vi "STARTUP.VI"() -> ()   [LabVIEW 2011]
uses:
  OIMENU.LLB/OIMenuItem1.ctl
panel:
  in  "ILM Setup Dialog":T1={"Go"=TRUE}
  in  "Array of VI's to open automatically on startup.\nCreate the list you require and save it using\nOperate-Make Current Values Default":cluster{"Library":string, "vi name":string}[](array[cluster])=[{"Library"="oimenu.llb", "vi name"="oimenu.vi"}]
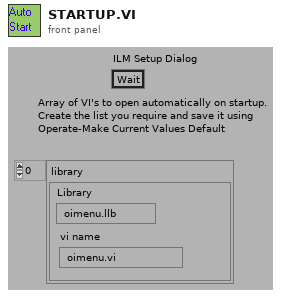
[diagram p1: front panel]
types:
  T1 = typedef "OIMenuItem1.ctl" = cluster{"Go":bool}
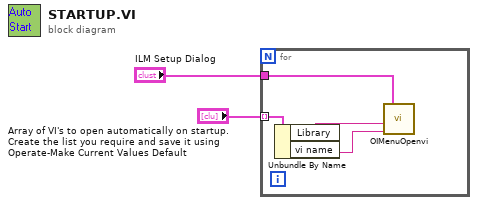
[diagram p0: block diagram]
diagram:
  n1 = for {
    tunnel: "Array of VI's to open automatically on startup.\nCreate the list you require and save it using\nOperate-Make Current Values Default" -> [w6] mode=indexing
    tunnel: "ILM Setup Dialog" -> [w3]
    n2 = Unbundle By Name(w6) -> ("Library"=w5:string, "vi name"=w4:string)
    n3 = call "OIMenuOpenvi.vi"("vi"=w4, "library"=w5, "ILM Setup Dialog"=w3) -> ()  [unwired: 5 in]
  }
